vi "Defer Panel Update.vi"(8 "error in (no error)":errorcluster, 10 "Defer Panel Updates(false)":bool, 11 "VI in":refnum<vi>) -> (0 "error out":errorcluster, 3 "VI  out":refnum<vi>)   [LabVIEW 2015]
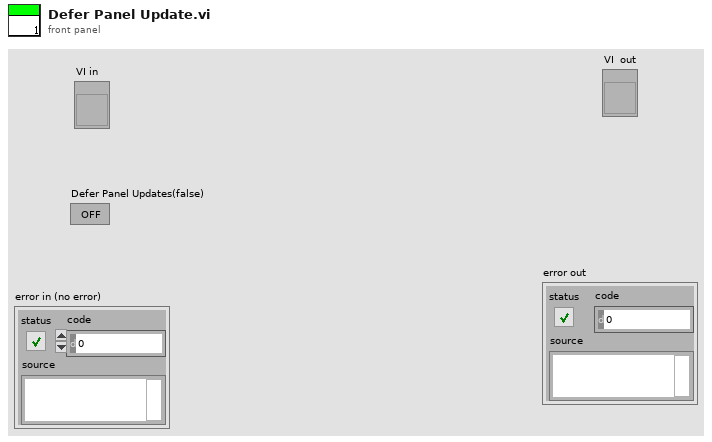
[diagram p1: front panel]
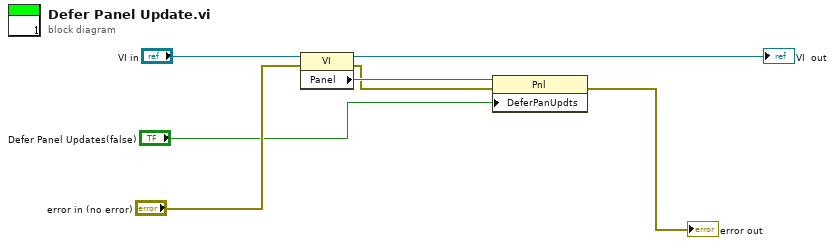
[diagram p0: block diagram]
diagram:
  n1 = property on="Property Node" class="VI"(reference="VI in", error in="error in (no error)") -> (reference out=→"VI  out":refnum<vi>, error out=w5:errorcluster, "Panel"=w6:refnum<vi>)
  n2 = property on="Property Node" class="Pnl"(reference=w6, error in=w5, "DeferPanUpdts"="Defer Panel Updates(false)") -> (error out=→"error out":errorcluster)  [unwired: 1 out]
